vi "Stop.vi"(8 "Error In":errorcluster, 11 "object in":refnum<class "IScope.lvclass">) -> (0 "Error Out":errorcluster, 3 "object out":refnum<class "IScope.lvclass">)   [LabVIEW 2023, in "IScope.lvclass"]
uses:
  IScope.lvclass
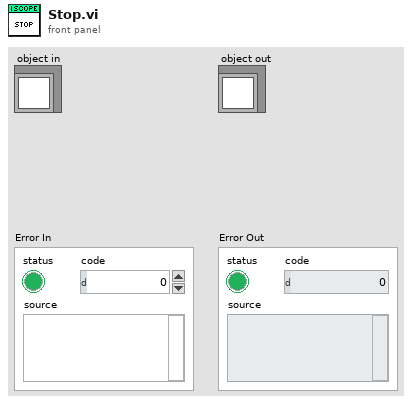
[diagram p1: front panel]
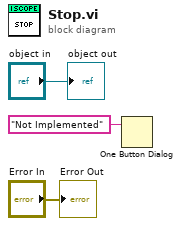
[diagram p0: block diagram]
diagram:
  n1 = One Button Dialog(message="Not Implemented") -> ()  [unwired: 1 in, 1 out]
  "Error Out" <- "Error In"
  "object out" <- "object in"
